vi "Initialize Attribute Channels.vi"(8 "error in (no error)":errorcluster, 10 "Number of Channels":i32, 11 "CS++DCPwrChannelData in":refnum<class "CS++DCPwrChannelData.lvclass">) -> (0 "error out":errorcluster, 3 "CS++DCPwrChannelData out":refnum<class "CS++DCPwrChannelData.lvclass">)   [LabVIEW 2016, in "CS++DCPwrGui.lvlib" / "CS++DCPwrChannelData.lvclass"]
uses:
  CS++DCPwrChannelData.lvclass
  CS++DCPwrChannelData.lvclass/CS++DCPwrChannelData.ctl
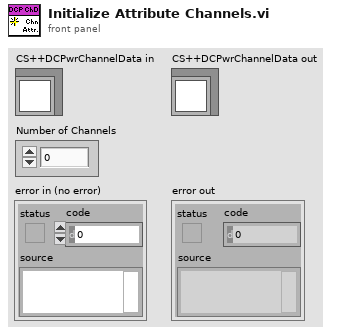
[diagram p1: front panel]
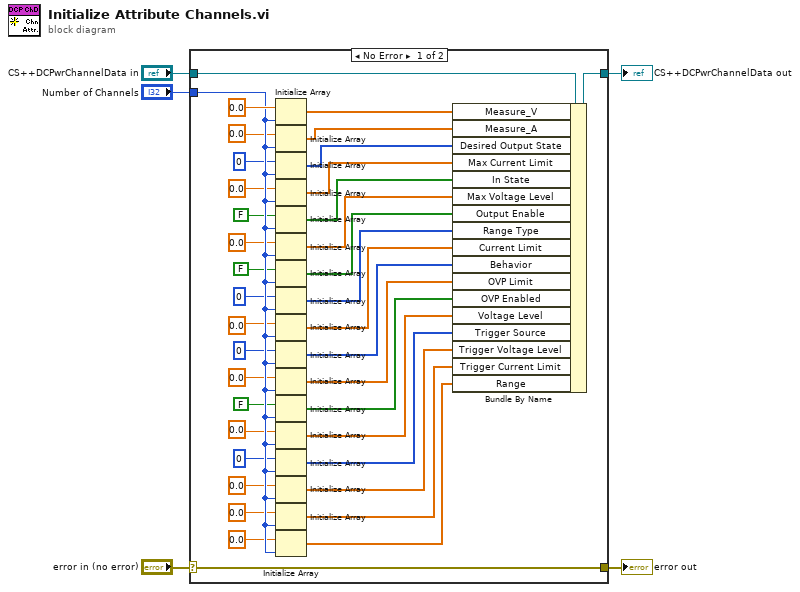
[diagram p0: block diagram]
diagram:
  n1 = case shown="No Error" "error in (no error)" {
    selector: "error in (no error)" -> [w43 w45]
    tunnel: [w43 w45] -> w4
    tunnel: [w41 w44] -> w2
    tunnel: "CS++DCPwrChannelData in" -> [w42 w44]
    tunnel: "Number of Channels" -> [w38 _]
    frame No Error {
      n2 = Initialize Array(dbl[unit] 0.0 ("measurement"), w38) -> (w39:dbl[unit][])
      n3 = Initialize Array(dbl[unit] 0.0 ("measurement"), w38) -> (w36:dbl[unit][])
      n4 = Initialize Array(0 ("output state (Constant Voltage)"), w38) -> (w34:i32[])
      n5 = Initialize Array(dbl[unit] 0.0 ("max current limit"), w38) -> (w32:dbl[unit][])
      n6 = Initialize Array(FALSE ("in state"), w38) -> (w30:bool[])
      n7 = Initialize Array(dbl[unit] 0.0 ("max voltage level"), w38) -> (w28:dbl[unit][])
      n8 = Initialize Array(FALSE ("enabled (true)"), w38) -> (w26:bool[])
      n9 = Initialize Array(0 ("range type (Voltage)"), w38) -> (w24:i32[])
      n10 = Initialize Array(dbl[unit] 0.0 ("limit (0.0 Amps)"), w38) -> (w22:dbl[unit][])
      n11 = Initialize Array(0 ("behavior (regulate)"), w38) -> (w20:i32[])
      n12 = Initialize Array(dbl[unit] 0.0 ("limit (0.0 Volts)"), w38) -> (w18:dbl[unit][])
      n13 = Initialize Array(FALSE ("enabled (true)"), w38) -> (w16:bool[])
      n14 = Initialize Array(dbl[unit] 0.0 ("level (0.0 Volts)"), w38) -> (w14:dbl[unit][])
      n15 = Initialize Array(0 ("source (Immediate)"), w38) -> (w12:i32[])
      n16 = Initialize Array(dbl[unit] 0.0 ("triggered level (0.0 Volts)"), w38) -> (w10:dbl[unit][])
      n17 = Initialize Array(dbl[unit] 0.0 ("triggered limit (0.0 Amps)"), w38) -> (w8:dbl[unit][])
      n18 = Initialize Array(0.0 ("range (0.0)"), w38) -> (w6:dbl[])
      n19 = Bundle By Name(cluster=w42, "Measure_V"=w39, "Measure_A"=w36, "Desired Output State"=w34, "Max Current Limit"=w32, "In State"=w30, "Max Voltage Level"=w28, "Output Enable"=w26, "Range Type"=w24, "Current Limit"=w22, "Behavior"=w20, "OVP Limit"=w18, "OVP Enabled"=w16, "Voltage Level"=w14, "Trigger Source"=w12, "Trigger Voltage Level"=w10, "Trigger Current Limit"=w8, "Range"=w6) -> (w41:refnum<class "CS++DCPwrChannelData.lvclass">)
    }
    frame Error {
    }
  }
  "error out" <- w4
  "CS++DCPwrChannelData out" <- w2
